vi "FGV Sanftanlauf Vortex.vi"(0 "Flanke":bool, 7 "Scantime Scanengine in ms":dbl, 9 "Perioden":u32, 11 "error in (no error)":errorcluster caption="Fehler (Eingang, kein Fehler)", 13 "Aktion":enum16{"init", "aktiv"}(ring)) -> (4 "Output":dbl, 15 "error out":errorcluster caption="Fehler (Ausgang)")   [LabVIEW 2020, in "Allgemein.lvlib"]
uses:
  Allgemein.lvlib
  Verwaltung/Verwaltung - cRIO.lvlib
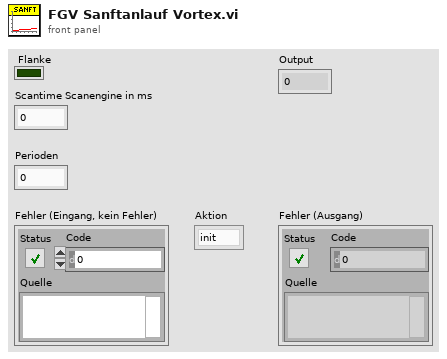
[diagram p1: front panel]
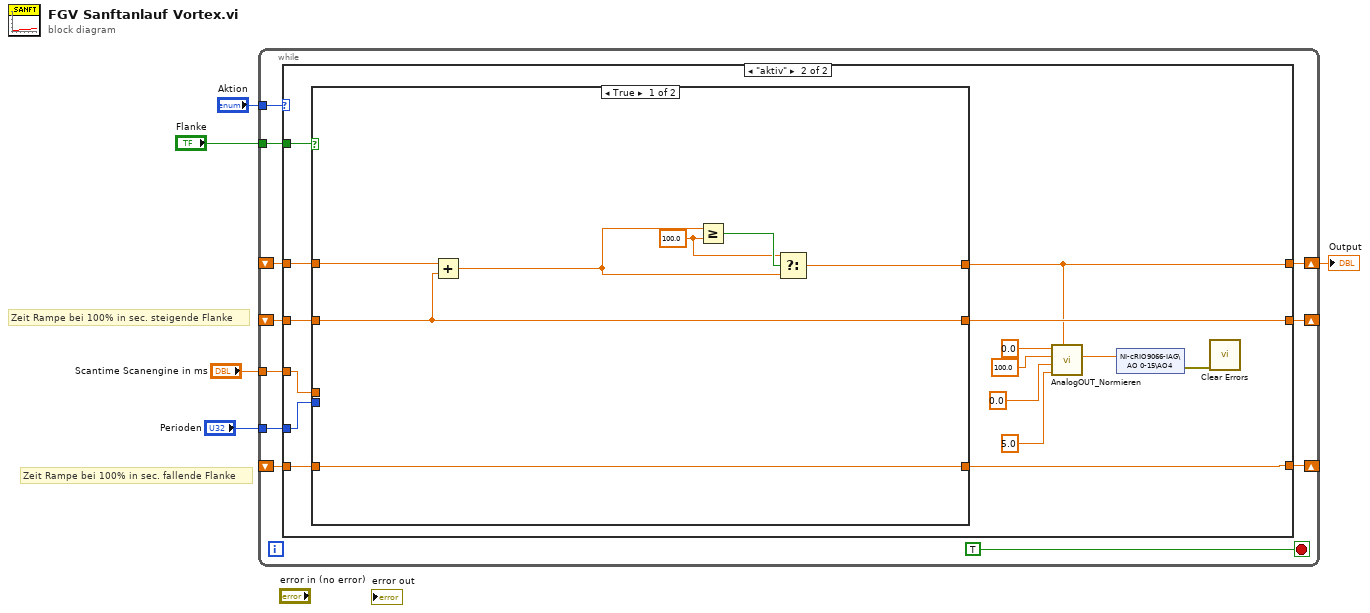
[diagram p0: block diagram]
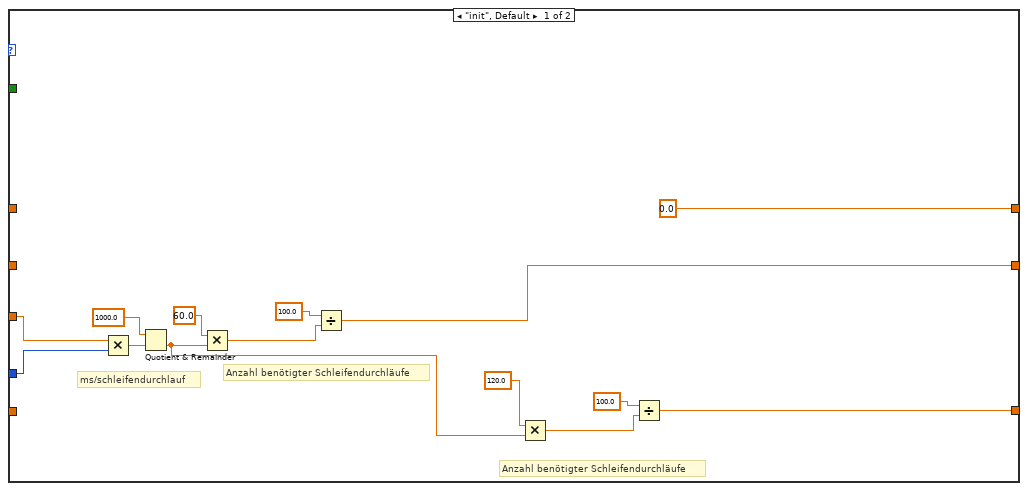
[diagram p2: hidden frame]
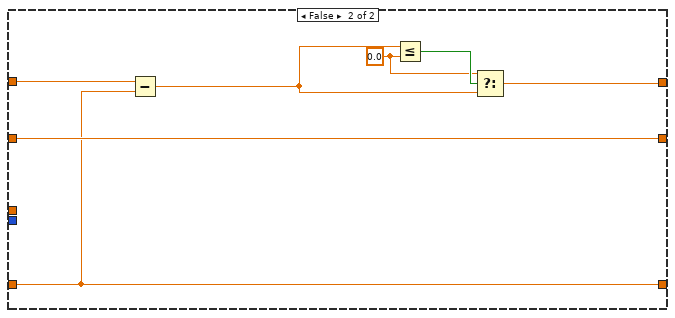
[diagram p3: hidden frame]
diagram:
  # "Zeit Rampe bei 100% in sec. fallende Flanke"
  # "Zeit Rampe bei 100% in sec. steigende Flanke"
  n1 = while {
    tunnel: "Flanke" -> [w15]
    tunnel: "Aktion" -> [w14]
    shift-right: [w13] -> w1
    shift-left: _ -> [w12]
    tunnel: "Scantime Scanengine in ms" -> [w10]
    tunnel: "Perioden" -> [w11]
    shift-right: [w9] -> _
    shift-left: _ -> [w8]
    shift-right: [w7] -> _
    shift-left: _ -> [w6]
    stop <- TRUE stop-if-true
    n2 = case shown="\"aktiv\"" w14 {
      tunnel: w15 -> [_ w45]
      tunnel: [0.0 w35] -> w13
      tunnel: w12 -> [_ w44]
      tunnel: w11 -> [w23 w42]
      tunnel: w10 -> [w24 w43]
      tunnel: [w22 w40] -> w9
      tunnel: w8 -> [_ w41]
      tunnel: [w17 w31] -> w7
      tunnel: w6 -> [_ w32]
      frame "init", Default {
        # "Anzahl benötigter Schleifendurchläufe"
        # "Anzahl benötigter Schleifendurchläufe"
        # "ms/schleifendurchlauf"
        n3 = Multiply(x=w24, y=w23) -> (x*y=w28:dbl)
        n4 = Quotient & Remainder(x=1000.0, y=w28) -> (floor(x/y)=w18:dbl)  [unwired: 1 out]
        n5 = Multiply(x=60.0, y=w18) -> (x*y=w25:dbl)
        n6 = Divide(x=100.0, y=w25) -> (x/y=w22:dbl)
        n7 = Multiply(x=120.0, y=w18) -> (x*y=w21:dbl)
        n8 = Divide(x=100.0, y=w21) -> (x/y=w17:dbl)
      }
      frame "aktiv" {
        n9 = case shown="True" w45 {
          tunnel: w44 -> [w52 w59]
          tunnel: w43 -> [_ _]
          tunnel: w42 -> [_ _]
          tunnel: w41 -> [w51 w58]
          tunnel: [w51 w58] -> w40
          tunnel: [w49 w56] -> w35
          tunnel: w32 -> [w46 w53]
          tunnel: [w46 w53] -> w31
          frame True {
            w47 = 100.0 ("y")
            n10 = Add(x=w52, y=w51) -> (x+y=w50:dbl)
            n11 = Greater Or Equal?(x=w50, y=w47) -> (x >= y?=w48:bool)
            n12 = Select(t=w47, s=w48, f=w50) -> (s? t:f=w49:dbl)
          }
          frame False {
            w54 = 0.0 ("y")
            n13 = Subtract(x=w59, y=w53) -> (x-y=w57:dbl)
            n14 = Less Or Equal?(x=w57, y=w54) -> (x <= y?=w55:bool)
            n15 = Select(t=w54, s=w55, f=w57) -> (s? t:f=w56:dbl)
          }
        }
        n16 = call "AnalogOUT_Normieren.vi"("Analogwert"=w35, "Obergrenze"=sgl 5.0, "Untergrenze"=sgl 0.0, "Max Analogwert"=sgl 100.0, "Min Analogwert"=sgl 0.0) -> ("Normierter Wert"=w33:sgl)  [unwired: 6 in]
        n17 = shared-variable "NI-cRIO9066-IAG\\AO 0-15\\AO4"(w33) -> (error out=w34:errorcluster)  [unwired: 1 in]
        n18 = call <vilib>:"Clear Errors.vi"("error in (no error)"=w34) -> ()  [unwired: 5 in, 2 out]
      }
    }
  }
  "Output" <- w1
